vi "Compute Saturated Gate Image Array.vi"(8 "error in (no error)":errorcluster, 10 "Saturation Parameters":T1, 11 "Gate Count Rate Array in":ext[](array[numeric])) -> (0 "error out":errorcluster, 3 "Saturated Gate Image Count Array out":ext[](array[numeric]))   [LabVIEW 2019]
doc: "Saturated recorded count rates for a detector with:\n\n- multiplicity p = 1 (e.g. SPAD)\n- counter capacity: q bits\n- number of gate accumulation per frame: L\n- number of frame accumulation: F"
uses:
  Photon-Counting Saturation Parameters.ctl
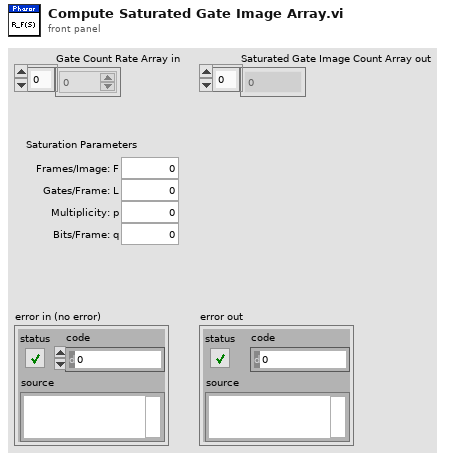
[diagram p1: front panel]
types:
  T1 = typedef "Photon-Counting Saturation Parameters.ctl" = cluster{"Frames/Image: F":i32, "Gates/Frame: L":i32, "Multiplicity: p":i32, "Bits/Frame: q":i32}
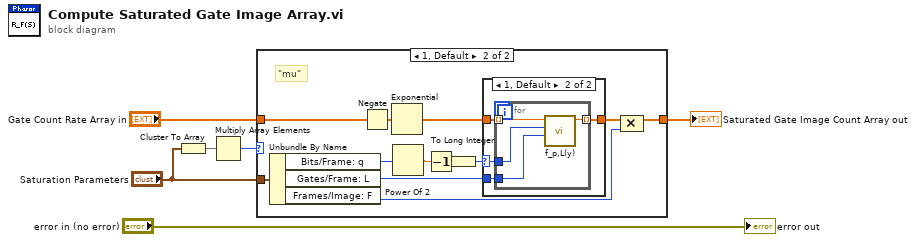
[diagram p0: block diagram]
diagram:
  n1 = Cluster To Array(cluster="Saturation Parameters") -> (array=w2:i32[])
  n2 = Multiply Array Elements(1:w2) -> (0:w1:i32)
  n3 = case shown="1, Default" w1 {
    tunnel: "Gate Count Rate Array in" -> [w7 w19]
    tunnel: [w7 w16] -> w5
    tunnel: "Saturation Parameters" -> [_ w15]
    frame 0 {
    }
    frame 1, Default {
      # "\"mu\""
      n4 = Unbundle By Name(w15) -> ("Bits/Frame: q"=w11:i32, "Gates/Frame: L"=w18:i32, "Frames/Image: F"=w12:i32)
      n5 = Negate(x=w19) -> (-x=w14:ext[])
      n6 = Exponential(1:w14) -> (0:w13:ext[])
      n7 = Power Of 2(x=w11) -> (2^x=w10:dbl)
      n8 = Decrement(x=w10) -> (x-1=w9:dbl)
      n9 = To Long Integer(number=w9) -> (32bit integer=w8:i32)
      n10 = case shown="1, Default" w8 {
        selector: w8 -> [_ w21]
        tunnel: w18 -> [_ w24]
        tunnel: [w20 w23] -> w17
        tunnel: w13 -> [w20 w22]
        frame ..0 {
        }
        frame 1, Default {
          n11 = for {
            tunnel: w22 -> [w28] mode=indexing
            tunnel: w21 -> [w27]
            tunnel: w24 -> [w26]
            tunnel: [w25] -> w23 mode=indexing
            n12 = call "f_p,L(y).vi"("L"=w26, "p"=w27, "y"=w28) -> ("f_p,L(y)"=w25:ext)  [unwired: 8 in]
          }
        }
      }
      n13 = Compound Arithmetic op=MULTIPLY(w17, w12) -> (w16:ext[])
    }
  }
  "Saturated Gate Image Count Array out" <- w5
  "error out" <- "error in (no error)"
